vi "Server_OpenHelp.vi"(6 "Server":path, 8 "error in (no error)":errorcluster) -> (0 "error out":errorcluster)   [LabVIEW 2020]
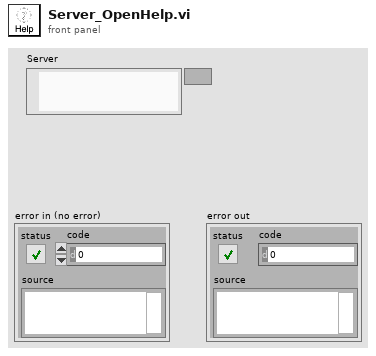
[diagram p1: front panel]
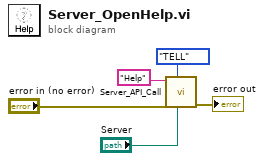
[diagram p0: block diagram]
diagram:
  n1 = call "Server_API_Call.vi"("Server"="Server", "Direction"=enum16{"ASK", "TELL"}."TELL", "error in (no error)"="error in (no error)", "cmd"="Help" ("url")) -> ("error out"=→"error out":errorcluster)  [unwired: 4 in, 3 out]
